vi "AddCONTSEQ.vi"(0 "VISA resource name":refnum<visa-resource-name>, 1 "Test Time (s)":string, 2 "Min Cont Limit (ohm)":string, 3 "Max Cont Limit (ohm)":string, 5 "error in (no error)":errorcluster, 6 "Sequence Number":string, 8 "Sequence Name":string) -> (14 "VISA resource name out":refnum<visa-resource-name>, 17 "Error Message":string, 18 "Error Code":i32, 19 "error out":errorcluster)   [LabVIEW 2010, in "VITREK V7X.lvlib"]
doc: "Add a new CONT test step into a sequence and save this sequence into the requested store number."
uses:
  VITREK V7X.lvlib
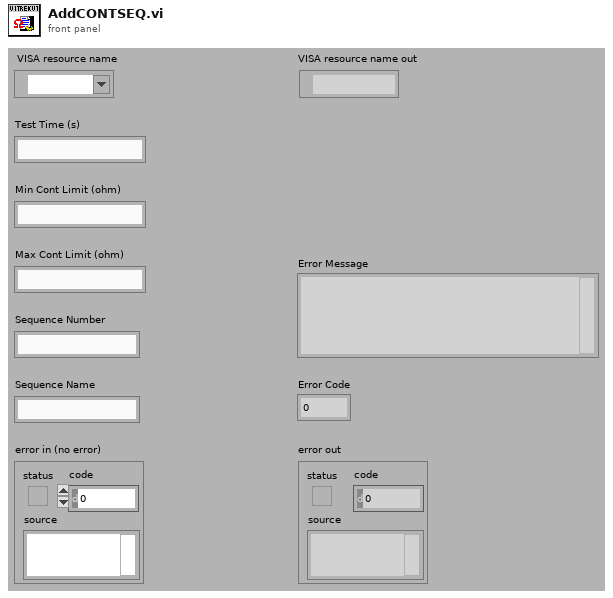
[diagram p1: front panel]
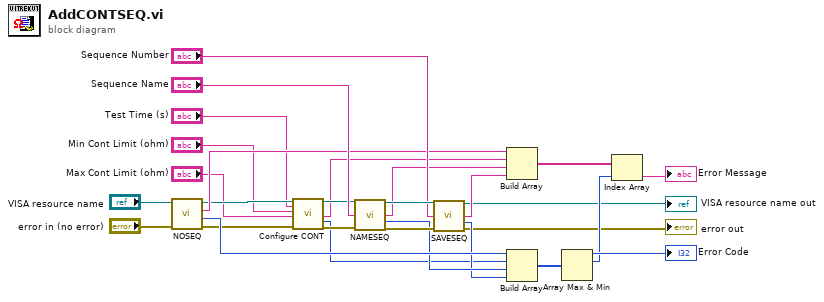
[diagram p0: block diagram]
diagram:
  n1 = call "NOSEQ.vi"("error in (no error)"="error in (no error)", "VISA resource name"="VISA resource name") -> ("error out"=w9:errorcluster, "Error Code"=w18:i32, "Error Message"=w15:string, "VISA resource name out"=w11:refnum<visa-resource-name>)  [unwired: 6 in]
  n2 = call "Configure CONT.vi"("VISA resource name"=w11, "Test Time (s)"="Test Time (s)", "Min Cont Limit (ohm)"="Min Cont Limit (ohm)", "Max Cont Limit (ohm)"="Max Cont Limit (ohm)", "error in (no error)"=w9) -> ("VISA resource name out"=w10:refnum<visa-resource-name>, "Error Message"=w4:string, "Error Code"=w3:i32, "error out"=w8:errorcluster)  [unwired: 10 in, 1 out]
  n3 = call "NAMESEQ.vi"("VISA resource name"=w10, "Sequence Name"="Sequence Name", "error in (no error)"=w8) -> ("VISA resource name out"=w25:refnum<visa-resource-name>, "Error Message"=w14:string, "Error Code"=w17:i32, "error out"=w26:errorcluster)  [unwired: 9 in]
  n4 = call "SAVESEQ.vi"("VISA resource name"=w25, "Sequence Number"="Sequence Number", "error in (no error)"=w26) -> ("VISA resource name out"=→"VISA resource name out":refnum<visa-resource-name>, "Error Message"=w13:string, "Error Code"=w16:i32, "error out"=→"error out":errorcluster)  [unwired: 9 in]
  n5 = Build Array(w15, w4, w14, w13) -> (w22:string[])
  n6 = Build Array(w18, w3, w17, w16) -> (w20:i32[])
  n7 = Array Max & Min(array=w20) -> (max value=→"Error Code":i32, max index (indices)=w12:i32)  [unwired: 2 out]
  n8 = Index Array(array=w22, index=w12) -> (element=→"Error Message":string)
